vi "Joystick Drive Control.vi"(10 "Arcade Drive?":bool, 11 "Cluster In":T11) -> ()   [LabVIEW 2018]
uses:
  <vilib>/Rock Robotics/WPI/MotorControl/WPI_MotorControlDeviceRef.ctl
  <vilib>/Rock Robotics/WPI/MotorControl/WPI_MotorControlType.ctl
  <vilib>/Rock Robotics/SystemInterfaces/DIO/FPGA_DIOPWMChannel.ctl
  <vilib>/Rock Robotics/WPI/PWM/WPI_PWMDeadband.ctl
  <vilib>/Rock Robotics/SystemInterfaces/DIO/FPGA_DIOChannel.ctl
  <vilib>/Rock Robotics/WPI/Joystick/WPI_JoystickDevRef.ctl
  <vilib>/Rock Robotics/WPI/Joystick/WPI_JoystickDeviceEnum.ctl
  <vilib>/Rock Robotics/WPI/DriverStation/WPI_DriverStationRobotMode2.ctl
  <vilib>/Rock Robotics/WPI/RobotDrive/WPI_RobotDriveDevRef.ctl
  Vision States.ctl
  <vilib>/Rock Robotics/WPI/ThirdParty/Phoenix-LabVIEW/Motor Controller/Controls/CTRE_Phoenix_MotorControl_ControlMode.ctl
  Robot Global Data.vi
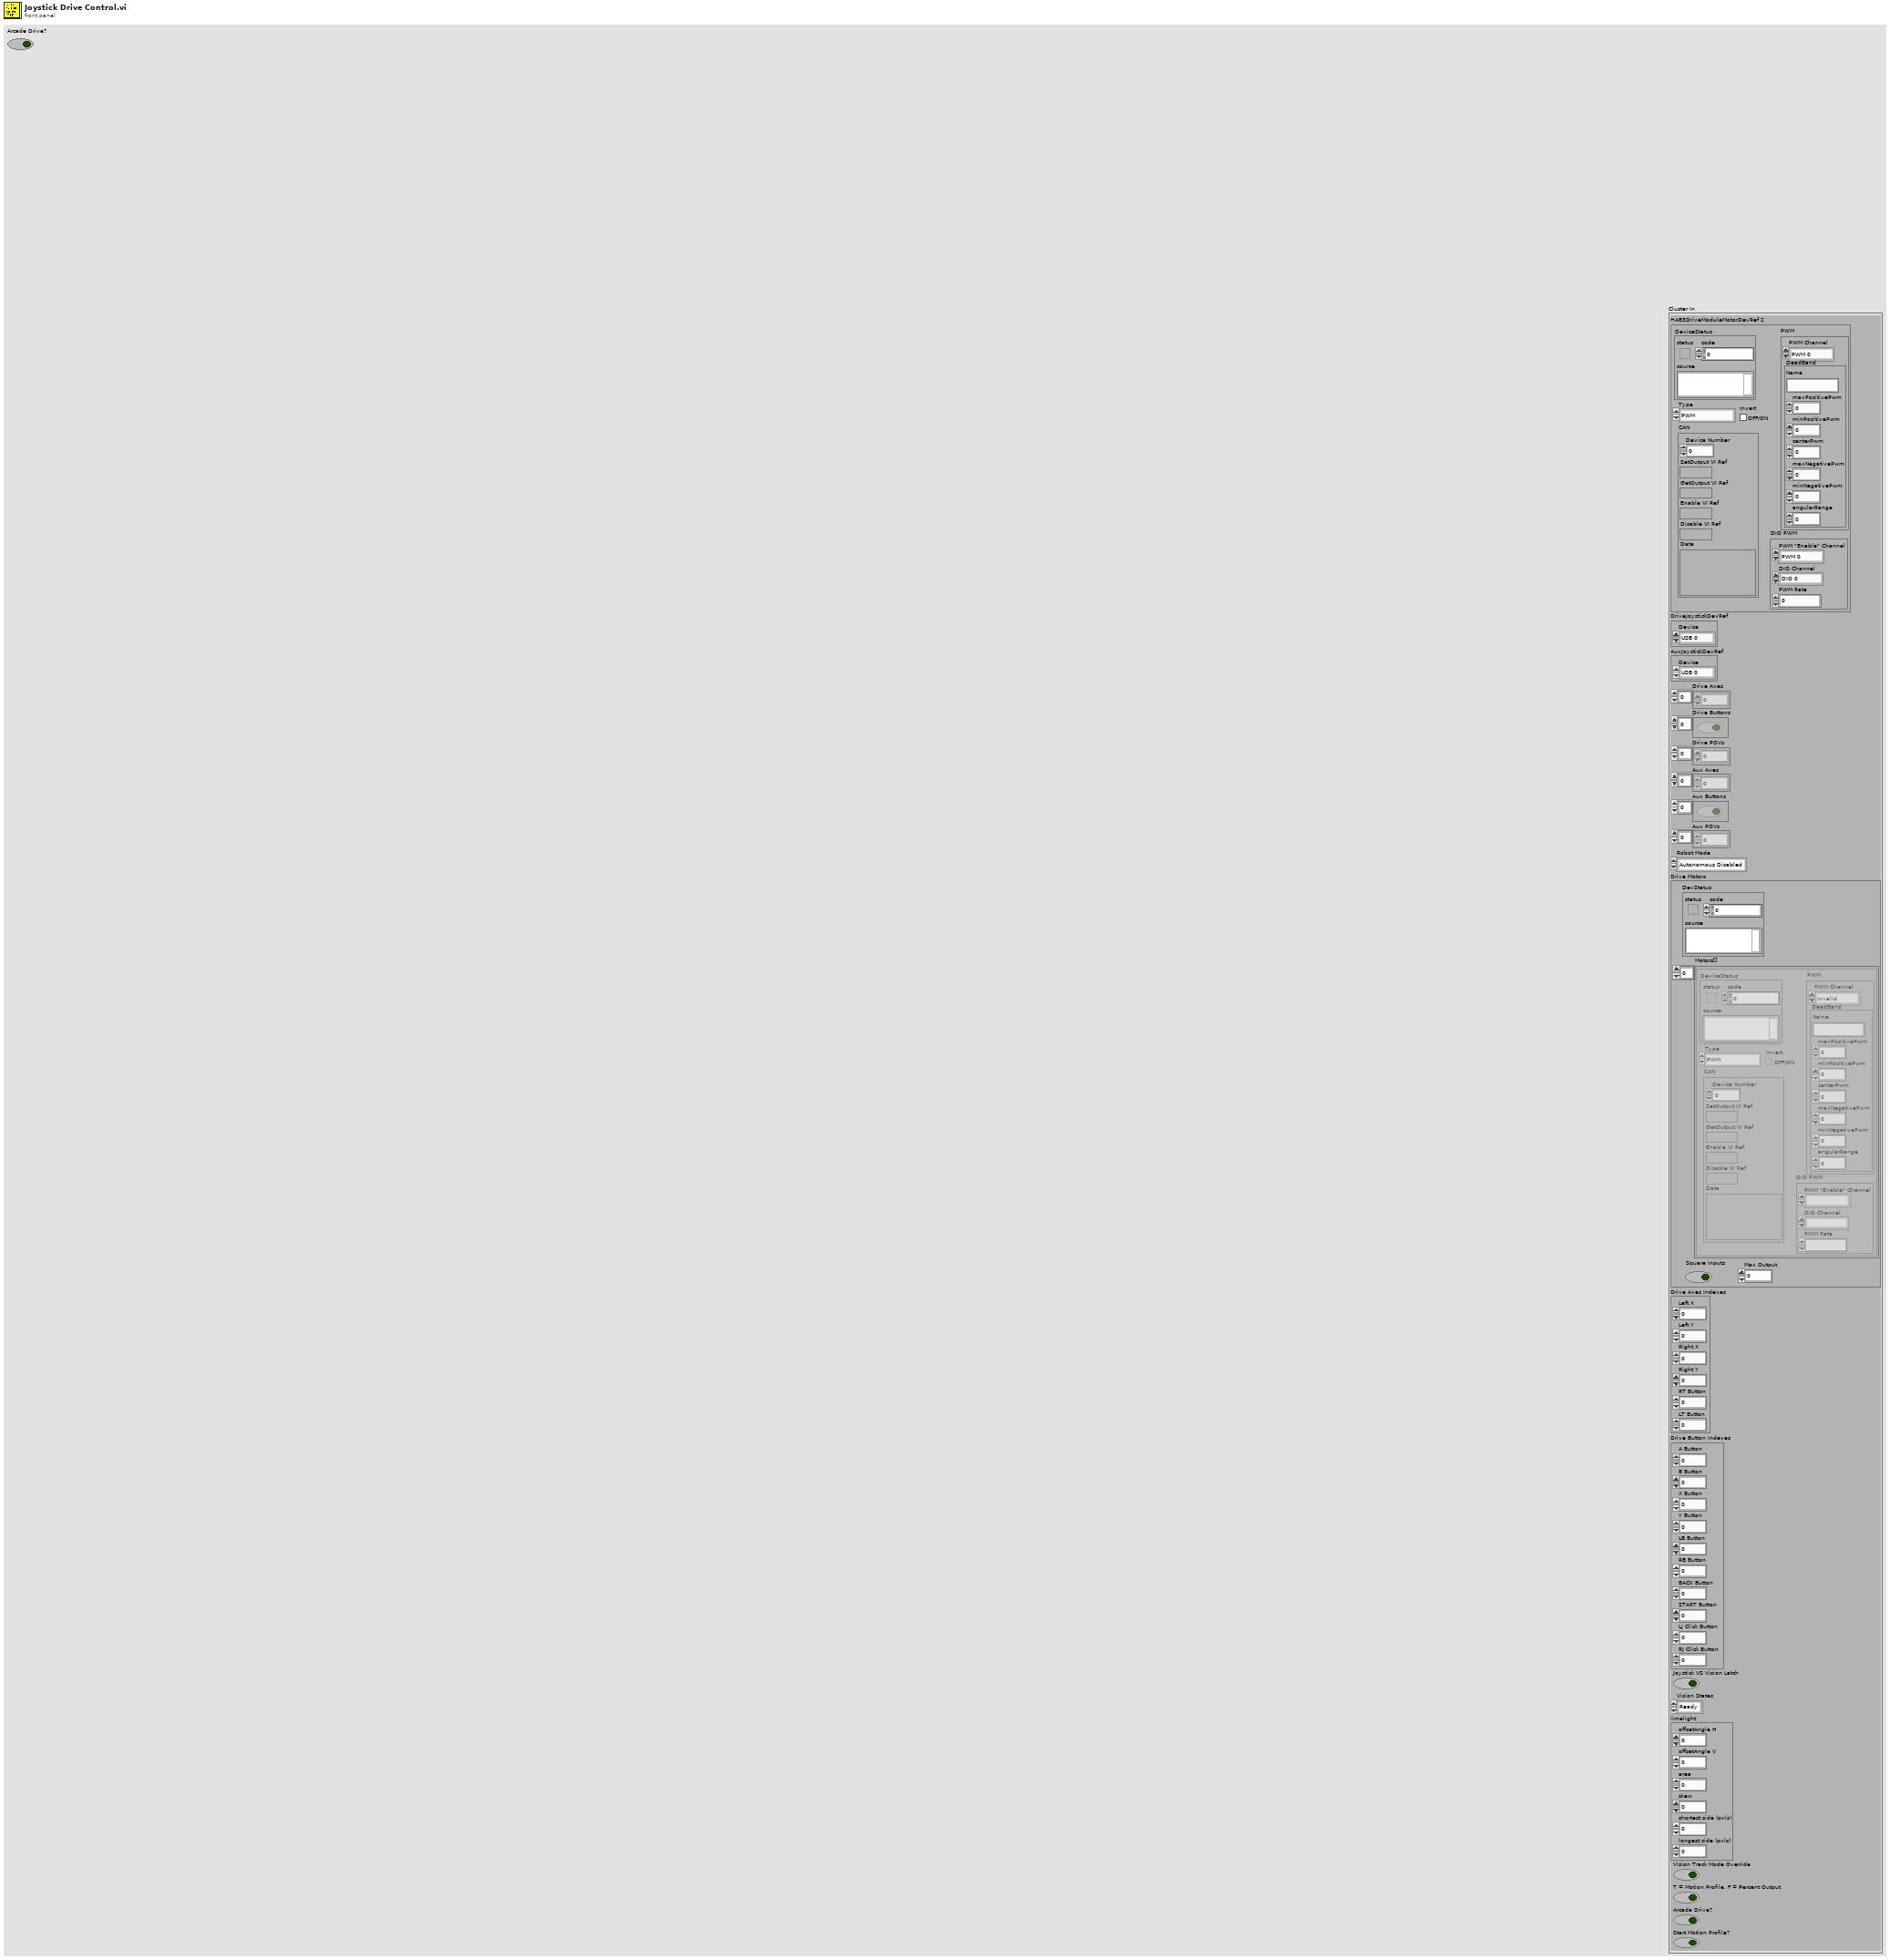
[diagram p1: front panel]
types:
  T1 = typedef "WPI_MotorControlDeviceRef.ctl" = cluster{"DeviceStatus":errorcluster, "Type":T2, "PWM":cluster{"PWM Channel":T3, "DeadBand":T4}, "CAN":cluster{"Device Number":u8, "SetOutput VI Ref":variant, "GetOutput VI Ref":variant, "Enable VI Ref":variant, "Disable VI Ref":variant, "Data":variant}, "Invert":bool, "DIO PWM":cluster{"PWM \"Enable\" Channel":T3, "DIOChannel":T5, "PWM Rate":dbl}}
  T2 = typedef "WPI_MotorControlType.ctl" = enum16{"PWM", "CAN", "DIO PWM"}
  T3 = typedef "FPGA_DIOPWMChannel.ctl" = enum8{"PWM 0", "PWM 1", "PWM 2", "PWM 3", "PWM 4", "PWM 5", "PWM 6", "PWM 7", "PWM 8", "PWM 9", "PWM MXP 0", "PWM MXP 1", "PWM MXP 2", "PWM MXP 3", "PWM MXP 4", "PWM MXP 5", "PWM MXP 6", "PWM MXP 7", "PWM MXP 8", "PWM MXP 9", "Invalid"}
  T4 = typedef "WPI_PWMDeadband.ctl" = cluster{"Name":string, "maxPositivePwm":i32, "minPositivePwm":i32, "centerPwm":i32, "maxNegativePwm":i32, "minNegativePwm":i32, "angularRange":u16}
  T5 = typedef "FPGA_DIOChannel.ctl" = enum8{"DIO 0", "DIO 1", "DIO 2", "DIO 3", "DIO 4", "DIO 5", "DIO 6", "DIO 7", "DIO 8", "DIO 9", "DIO MXP 0", "DIO MXP 1", "DIO MXP 2", "DIO MXP 3", "DIO MXP 4", "DIO MXP 5", "DIO MXP 6", "DIO MXP 7", "DIO MXP 8", "DIO MXP 9", "DIO MXP 10", "DIO MXP 11", "DIO MXP 12", "DIO MXP 13", "DIO MXP 14", "DIO MXP 15", "SPI Port CS1", "SPI Port CS2", "SPI Port CS3", "SPI Port MISO", "SPI Port MOSI", "Invalid"}
  T6 = typedef "WPI_JoystickDevRef.ctl" = cluster{"Device":T7}
  T7 = typedef "WPI_JoystickDeviceEnum.ctl" = enum16{"USB 0", "USB 1", "USB 2", "USB 3", "USB 4", "USB 5"}
  T8 = typedef "WPI_DriverStationRobotMode2.ctl" = enum16{"Autonomous Disabled", "Autonomous Enabled", "Teleop Disabled", "Teleop Enabled", "Disconnected", "Finish", "Test Disabled", "Test Enabled", "Emergency Stopped"}
  T9 = typedef "WPI_RobotDriveDevRef.ctl" = cluster{"DevStatus":errorcluster, "Motors[]":T1[], "Square Inputs":bool, "Max Output":dbl}
  T10 = typedef "Vision States.ctl" = enum16{"Ready", "Forward Until Target at Edge", "Vision Track"}
  T11 = cluster{"HAB3DriveModuleMotorDevRef 2":T1, "DriveJoystickDevRef":T6, "AuxJoystickDevRef":T6, "Drive Axes":dbl[], "Drive Buttons":bool[], "Drive POVs":i16[], "Aux Axes":dbl[], "Aux Buttons":bool[], "Aux POVs":i16[], "Robot Mode":T8, "Drive Motors":T9, "Drive Axes Indexes":cluster{"Left X":i32, "Left Y":i32, "Right X":i32, "Right Y":i32, "RT Button":i32, "LT Button":i32}, "Drive Button Indexes":cluster{"A Button":i32, "B Button":i32, "X Button":i32, "Y Button":i32, "LB Button":i32, "RB Button":i32, "BACK Button":i32, "START Button":i32, "LJ Click Button":i32, "RJ Click Button":i32}, "Joystick VS Vision Latch":bool, "Vision States":T10, "limelight":cluster{"offsetAngle H":dbl, "offsetAngle V":dbl, "area":dbl, "skew":dbl, "shortest side (pxls)":dbl, "longest side (pxls)":dbl}, "Vision Track Mode Override":bool, "T = Motion Profile, F = Percent Output":bool, "Arcade Drive?":bool, "Start Motion Profile?":bool}
  T12 = typedef "CTRE_Phoenix_MotorControl_ControlMode.ctl" = u16
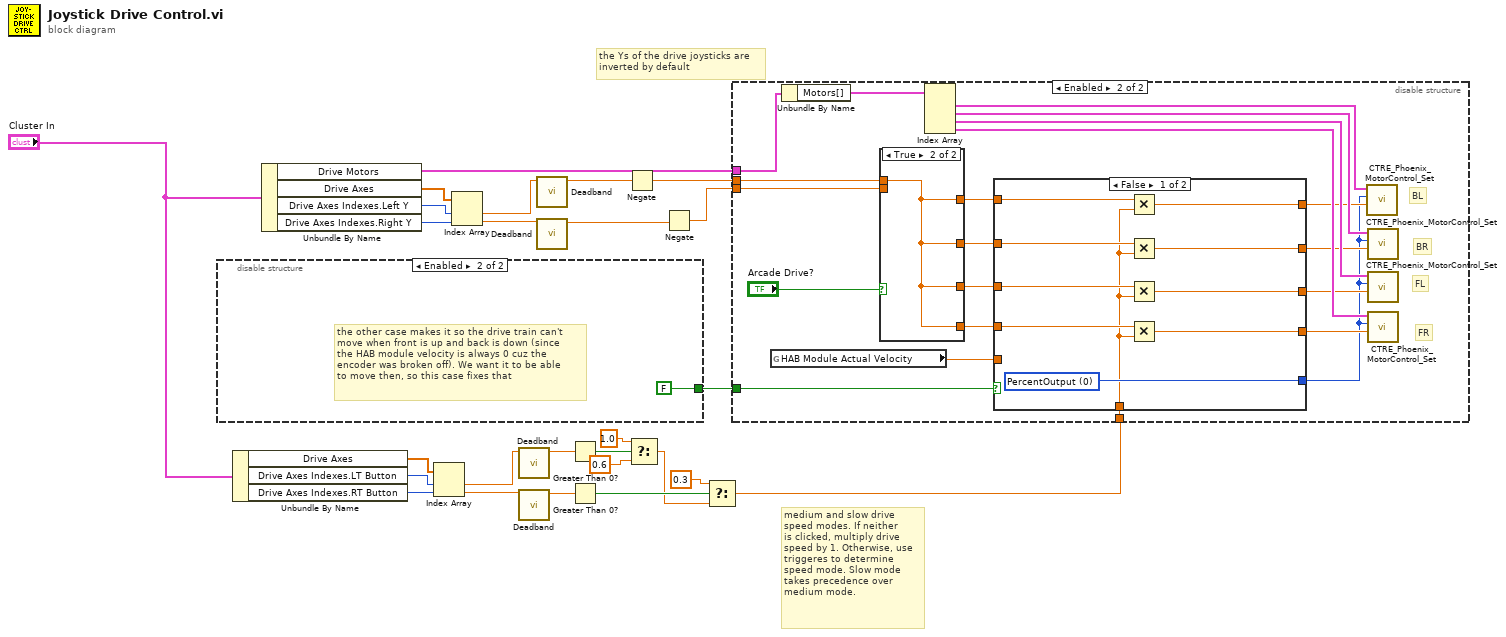
[diagram p0: block diagram]
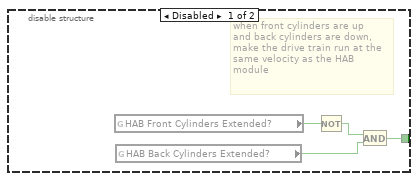
[diagram p2: hidden frame]
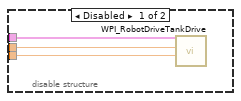
[diagram p3: hidden frame]
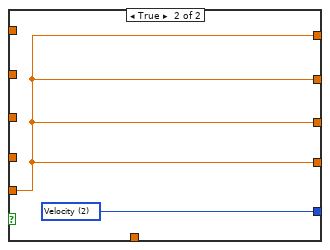
[diagram p5: hidden frame]
diagram:
  # "medium and slow drive\nspeed modes. If neither\nis clicked, multiply drive\nspeed by 1. Otherwise, use\ntriggeres to determine \nspeed mode. Slow mode\ntakes precedence over \nmedium mode."
  # "the Ys of the drive joysticks are \ninverted by default"
  n1 = disable-structure shown="Enabled" {
    disable-tunnel: [w28 FALSE] -> w16
    frame Disabled {
      # "when front cylinders are up\nand back cylinders are down,\nmake the drive train run at the\nsame velocity as the HAB \nmodule"
      n2 = global read "Robot Global Data.vi" "HAB Front Cylinders Extended?"() -> (w30:bool)
      n3 = global read "Robot Global Data.vi" "HAB Back Cylinders Extended?"() -> (w27:bool)
      n4 = Not(x=w30) -> (.not. x?=w29:bool)
      n5 = And(x=w29, y=w27) -> (x .and. y?=w28:bool)
    }
    frame Enabled {
      # "the other case makes it so the drive train can't\nmove when front is up and back is down (since\nthe HAB module velocity is always 0 cuz the \nencoder was broken off). We want it to be able \nto move then, so this case fixes that"
    }
  }
  n6 = Unbundle By Name("Cluster In") -> ("Drive Axes"=w12:dbl[], "Drive Axes Indexes.LT Button"=w13:i32, "Drive Axes Indexes.RT Button"=w14:i32)
  n7 = Unbundle By Name("Cluster In") -> ("Drive Motors"=w17:T9, "Drive Axes"=w18:dbl[], "Drive Axes Indexes.Left Y"=w19:i32, "Drive Axes Indexes.Right Y"=w20:i32)
  n8 = Index Array(array=w12, index #1=w13, index #2=w14) -> (element #1=w11:dbl, element #2=w15:dbl)
  n9 = Index Array(array=w18, index #1=w19, index #2=w20) -> (element #1=w23:dbl, element #2=w24:dbl)
  n10 = call "Deadband.vi"("Input"=w11) -> ("Output"=w10:dbl)  [unwired: 10 in]
  n11 = call "Deadband.vi"("Input"=w15) -> ("Output"=w9:dbl)  [unwired: 10 in]
  n12 = call "Deadband.vi"("Input"=w23) -> ("Output"=w26:dbl)  [unwired: 10 in]
  n13 = call "Deadband.vi"("Input"=w24) -> ("Output"=w25:dbl)  [unwired: 10 in]
  n14 = Greater Than 0?(x=w10) -> (x > 0?=w7:bool)
  n15 = Greater Than 0?(x=w9) -> (x > 0?=w8:bool)
  n16 = Negate(x=w26) -> (-x=w22:dbl)
  n17 = Select(t=1.0, s=w7, f=0.6) -> (s? t:f=w4:dbl)
  n18 = Negate(x=w25) -> (-x=w21:dbl)
  n19 = Select(t=0.3, s=w8, f=w4) -> (s? t:f=w2:dbl)
  n20 = disable-structure shown="Enabled" {
    disable-tunnel: w22 -> [w34 w39]
    disable-tunnel: w21 -> [w33 w37]
    disable-tunnel: w17 -> [w32 w55]
    disable-tunnel: w16 -> [_ w45]
    disable-tunnel: w2 -> [_ w42]
    frame Disabled {
      n21 = call <vilib>:"WPI_RobotDriveTankDrive.vi"("Right axis value"=w33, "Left axis value"=w34, "RobotDriveDevRef"=w32) -> ()  [unwired: 6 in, 3 out]
    }
    frame Enabled {
      # "FR"
      # "FL"
      # "BR"
      # "BL"
      n22 = global read "Robot Global Data.vi" "HAB Module Actual Velocity"() -> (w44:dbl)
      n23 = Unbundle By Name(w55) -> ("Motors[]"=w54:T1[])
      n24 = case shown="True" "Arcade Drive?" {
        tunnel: [w57 w58] -> w40
        tunnel: w39 -> [w57 w58]
        tunnel: [w56 w58] -> w38
        tunnel: w37 -> [w56 _]
        tunnel: [w57 w58] -> w36
        tunnel: [w56 w58] -> w35
        frame False {
        }
        frame True {
        }
      }
      n25 = Index Array(array=w54) -> (element #1=w53:T1, element #2=w50:T1, element #3=w52:T1, element #4=w51:T1)  [unwired: 4 in]
      n26 = case shown="False" w45 {
        tunnel: w40 -> [w68 _]
        tunnel: [w60 w70] -> w49
        tunnel: w35 -> [w65 _]
        tunnel: [w63 w70] -> w48
        tunnel: w36 -> [w66 _]
        tunnel: [w62 w70] -> w47
        tunnel: w38 -> [w67 _]
        tunnel: [w61 w70] -> w46
        tunnel: w44 -> [_ w70]
        tunnel: [w64 w69] -> w43
        tunnel: w42 -> [w59 _]
        frame False {
          w64 = T12 0 items=["PercentOutput"=0, "Position"=1, "Velocity"=2, "Current"=3, "Follower"=5, "MotionProfile"=6, "MotionMagic"=7, "MotionProfileArc"=10, "Disabled"=15] ("Control Mode")
          n27 = Multiply(x=w68, y=w59) -> (x*y=w60:dbl)
          n28 = Multiply(x=w67, y=w59) -> (x*y=w61:dbl)
          n29 = Multiply(x=w66, y=w59) -> (x*y=w62:dbl)
          n30 = Multiply(x=w65, y=w59) -> (x*y=w63:dbl)
        }
        frame True {
          w69 = T12 2 items=["PercentOutput"=0, "Position"=1, "Velocity"=2, "Current"=3, "Follower"=5, "MotionProfile"=6, "MotionMagic"=7, "MotionProfileArc"=10, "Disabled"=15] ("Control Mode")
        }
      }
      n31 = call <vilib>:"CTRE_Phoenix_MotorControl_Set.vi"("Output"=w49, "Control Mode"=w43, "PhoenixMotorControlDevRef"=w53) -> ()  [unwired: 7 in, 2 out]
      n32 = call <vilib>:"CTRE_Phoenix_MotorControl_Set.vi"("Output"=w46, "Control Mode"=w43, "PhoenixMotorControlDevRef"=w50) -> ()  [unwired: 7 in, 2 out]
      n33 = call <vilib>:"CTRE_Phoenix_MotorControl_Set.vi"("Output"=w47, "Control Mode"=w43, "PhoenixMotorControlDevRef"=w52) -> ()  [unwired: 7 in, 2 out]
      n34 = call <vilib>:"CTRE_Phoenix_MotorControl_Set.vi"("Output"=w48, "Control Mode"=w43, "PhoenixMotorControlDevRef"=w51) -> ()  [unwired: 7 in, 2 out]
    }
  }
